vi "bit-shift filter.vi"(7 "filterConstant":i16=-4 min=-6 max=0, 11 "newValue":sgl) -> (3 "filteredValue":sgl)   [LabVIEW 2018]
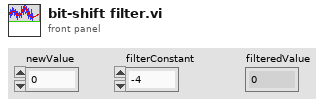
[diagram p1: front panel]
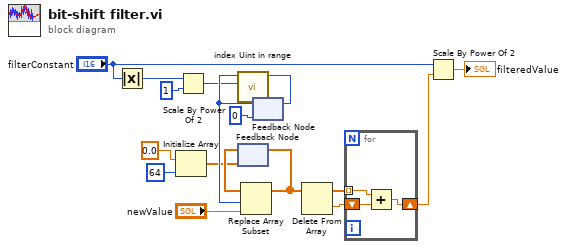
[diagram p0: block diagram]
diagram:
  n1 = Absolute Value(x="filterConstant") -> (abs(x)=w8:i16)
  n2 = Initialize Array(sgl 0.0 ("element"), 64 ("dimension size")) -> (w11:sgl[])
  n3 = Scale By Power Of 2(n=w8, x=1 ("dimension size")) -> (x*2^n=w6:i32)
  n4 = feedback #1(w11) -> (w14:sgl[])
  n5 = feedback #2(u8 0 ("new index")) -> (w15:u8)
  n6 = call "index Uint in range.vi"("limit"=w6, "index"=w15) -> ("new index"=w16:u8)  [unwired: 9 in]
  n7 = Replace Array Subset(array=w14, new element="newValue", index=w15) -> (w4:sgl[])
  n8 = feedback-in #1(w4) -> ()
  n9 = feedback-in #2(w16) -> ()
  n10 = Delete From Array(array=w4) -> (deleted portion=w2:sgl, array with subset deleted=w3:sgl[])  [unwired: 2 in]
  n11 = for {
    tunnel: w3 -> [w19] mode=indexing
    shift-right: [w18] -> w1
    shift-left: w2 -> [w20]
    n12 = Add(x=w19, y=w20) -> (x+y=w18:sgl)
  }
  n13 = Scale By Power Of 2(n="filterConstant", x=w1) -> (x*2^n=→"filteredValue":sgl)
